vi "Read Holding Registers.vi"(8 "error in (no error)":errorcluster, 9 "number of holding registers":u16, 10 "starting address":u16, 11 "Modbus master in":refnum<class "Network Master.lvclass">) -> (0 "error out":errorcluster, 2 "register values":u16[](array[numeric]), 3 "Modbus master out":refnum<class "Network Master.lvclass">)   [LabVIEW 2021, in "Network Master.lvclass"]
doc: "Reads values from contiguous holding registers. The maximum number of holding registers this VI can read is 125."
uses:
  Network Master.lvclass
  D:/my_projects/projects/Algorithms/Labview/21/Modbus_v121c/Network Protocol/Network Protocol.lvclass
  Modbus Data Unit/Modbus Data Unit.lvclass/Modbus Data Unit.ctl
  Network Protocol.lvclass/Network Protocol.ctl
  Network Master.lvclass/Network Master.ctl
  Modbus Data Unit/Construct PDU.vi
  Utility/Bytes to U16s.vi
  Master Function Definition/Function code mismatch error.vi
  Data Model/Error Generator.vi
  Modbus Data Unit/Deconstruct PDU.vi
  Read Transmission Data Unit.vi
  Modbus Data Unit/Modbus Data Unit.lvclass
  Transmission Data Unit/Transmission Data Unit.lvclass
  Master Function Definition/Master Function Definition.lvclass
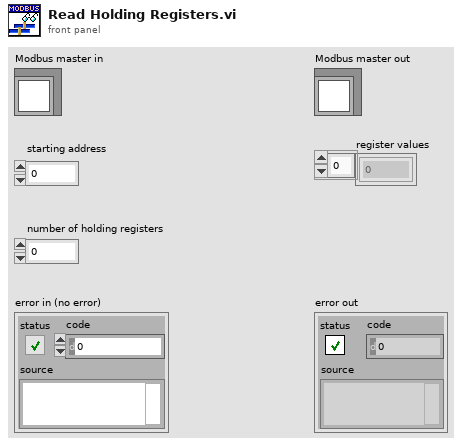
[diagram p1: front panel]
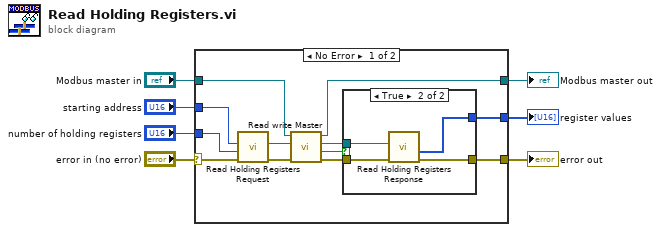
[diagram p0: block diagram]
diagram:
  n1 = case shown="No Error" "error in (no error)" {
    selector: "error in (no error)" -> [w8 w25]
    tunnel: "number of holding registers" -> [w15 _]
    tunnel: "starting address" -> [w16 _]
    tunnel: "Modbus master in" -> [w9 w26]
    tunnel: [w10 w26] -> w3
    tunnel: [w17 w25] -> w2
    tunnel: [w14 _] -> w1
    frame No Error {
      n2 = call "Read Holding Registers Request.vi"("error in"=w8, "Number of Registers"=w15, "Starting Address"=w16) -> ("error out"=w18:errorcluster, "modbus data unit out"=w11:refnum<class "Modbus Data Unit.lvclass">)  [unwired: 7 in]
      n3 = call "Read write Master.vi"("error in (no error)"=w18, "Modbus data unit in"=w11, "Modbus master in"=w9) -> ("error out"=w19:errorcluster, "PDU valid?"=w13:bool, "Modbus data unit out"=w12:refnum<class "Modbus Data Unit.lvclass">, "Modbus master out"=w10:refnum<class "Network Master.lvclass">)  [unwired: 5 in]
      n4 = case shown="True" w13 {
        tunnel: w19 -> [w20 w24]
        tunnel: [w20 w23] -> w17
        tunnel: [_ w22] -> w14
        tunnel: w12 -> [_ w21]
        frame False {
        }
        frame True {
          n5 = call "Read Holding Registers Response.vi"("error in"=w24, "modbus data unit in"=w21) -> ("error out"=w23:errorcluster, "Register Values"=w22:u16[])  [unwired: 7 in, 1 out]
        }
      }
    }
    frame Error {
    }
  }
  "Modbus master out" <- w3
  "error out" <- w2
  "register values" <- w1
